vi "Client Complete Streaming Call.vi"(8 "error in":errorcluster, 10 "Cancel All Reads (F)":bool, 11 "Call ID in":T2) -> (0 "error out":errorcluster, 1 "errorDetails":T1)   [LabVIEW 2019, in "grpc-lvsupport.lvlib"]
doc: "Set \"Cancel All Reads\" to true to end all pending reads and ignore any outstanding data from server that hasn't been read yet. If this setting is false, all server data must be read before the client can close the stream."
uses:
  grpc-lvsupport.lvlib
  grpcId.ctl
  Any.ctl
  <vilib>/Utility/error.llb/Error Cluster From Error Code.vi
  <resource>/labview_grpc_server.dll
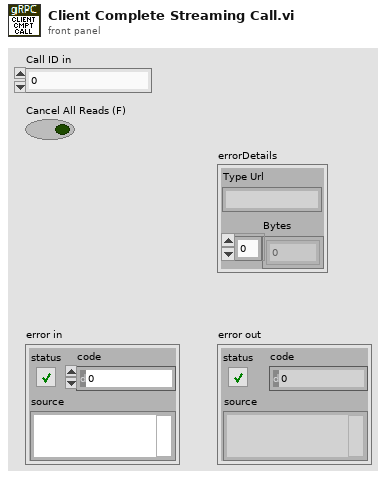
[diagram p1: front panel]
types:
  T1 = typedef "grpc-lvsupport.lvlib/Any.ctl" = cluster{"Type Url":string, "Bytes":u8[]}
  T2 = typedef "grpc-lvsupport.lvlib/grpcId.ctl" = u64
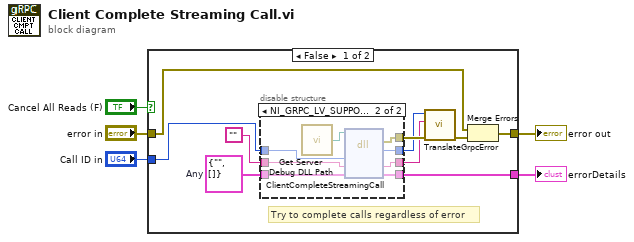
[diagram p0: block diagram]
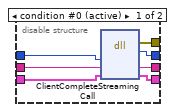
[diagram p2: hidden frame]
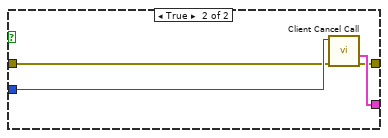
[diagram p3: hidden frame]
diagram:
  n1 = case shown="False" "Cancel All Reads (F)" {
    tunnel: "Call ID in" -> [w15 w34]
    tunnel: [w14 w33] -> w4
    tunnel: [w7 w32] -> w1
    tunnel: "error in" -> [w6 w31]
    frame False {
      w12 = T1 {"Type Url"="", "Bytes"=[]}  # Any
      # "Try to complete calls regardless of error"
      n2 = disable-structure shown="NI_GRPC_LV_SUPPORT_DEBUG==True&&RUN_TIME_ENGINE==False" {
        disable-tunnel: [w22 w30] -> w11
        disable-tunnel: w15 -> [w21 w29]
        disable-tunnel: w12 -> [w20 w28]
        disable-tunnel: [w19 w27] -> w14
        disable-tunnel: [w18 w26] -> w10
        disable-tunnel: [w17 w25] -> w9
        disable-tunnel: "" -> [w16 w24]
        frame condition #0 (active) {
          n3 = dll-call lib="C:/Program Files (x86)/National Instruments/LabVIEW 2024/resource/labview_grpc_server.*" fn="ClientCompleteStreamingCall"("ClientId"=w21, "errorMessage"=w16, "errorDetails"=w20) -> (error out=w22:errorcluster, "return type"=w17:i32, "errorMessage"=w18:string, "errorDetails"=w19:T1)  [unwired: 4 in, 1 out]
        }
        frame condition #1 {
          n4 = call "Get Server Debug DLL Path.vi"() -> ("DLL Path"=w23:path)
          n5 = dll-call lib="?" fn="ClientCompleteStreamingCall"(path in=w23, "ClientId"=w29, "errorMessage"=w24, "errorDetails"=w28) -> (error out=w30:errorcluster, "return type"=w25:i32, "errorMessage"=w26:string, "errorDetails"=w27:T1)  [unwired: 3 in, 1 out]
        }
      }
      n6 = call "TranslateGrpcError.vi"("error in"=w11, "Error Message"=w10, "Error Code"=w9) -> ("error out"=w8:errorcluster)  [unwired: 8 in]
      n7 = Merge Errors(w6, w8) -> (w7:errorcluster)
    }
    frame True {
      n8 = call "Client Cancel Call.vi"("error in"=w31, "Call ID in"=w34) -> ("error out"=w32:errorcluster, "errorDetails"=w33:T1)  [unwired: 7 in, 1 out]
    }
  }
  "error out" <- w1
  "errorDetails" <- w4
